vi "exec.vi"(8 "error in (no error)":errorcluster, 10 "context":refnum<class "IContextThisComponent.lvclass">, 11 "Enable in":refnum<class "Enable.lvclass">) -> (0 "error out":errorcluster, 2 "context 2":refnum<class "IContextThisComponent.lvclass">, 3 "Enable out":refnum<class "Enable.lvclass">)   [LabVIEW 2016, in "Commands.lvlib" / "Enable.lvclass"]
uses:
  Enable.lvclass
  IContextThisComponent/IContextThisComponent.lvclass
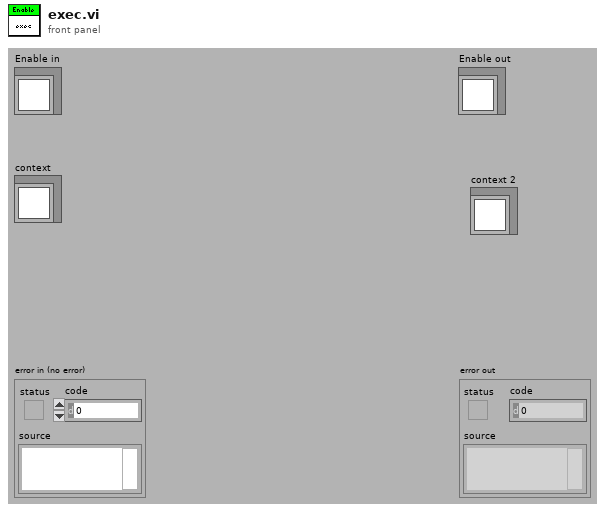
[diagram p1: front panel]
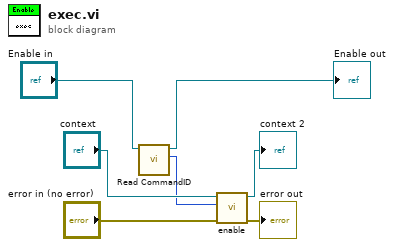
[diagram p0: block diagram]
diagram:
  n1 = call-dynamic "Read CommandID.vi"("Command in"="Enable in") -> ("CommandID"=w2:i32, "Command out"=→"Enable out":refnum<class "Enable.lvclass">)  [unwired: 8 in, 1 out]
  n2 = call-dynamic "enable.vi"("error in (no error)"="error in (no error)", "CommandID"=w2, "IContextThisComponent in"="context") -> ("error out"=→"error out":errorcluster, "IContextThisComponent out"=→"context 2":refnum<class "IContextThisComponent.lvclass">)  [unwired: 7 in]
